vi "Check Adapter.vi"(8 "error in (no error)":errorcluster, 11 "Execution Service":refnum<class "Execution Service.lvclass">) -> (0 "error out":errorcluster, 3 "Adapter Loaded":bool)   [LabVIEW 2026, in "Execution Service.lvclass"]
uses:
  Execution Service.lvclass
  Execution Service.lvclass/Execution Service.ctl
  Interfaces/I Execution Adapter/I Execution Adapter.lvclass
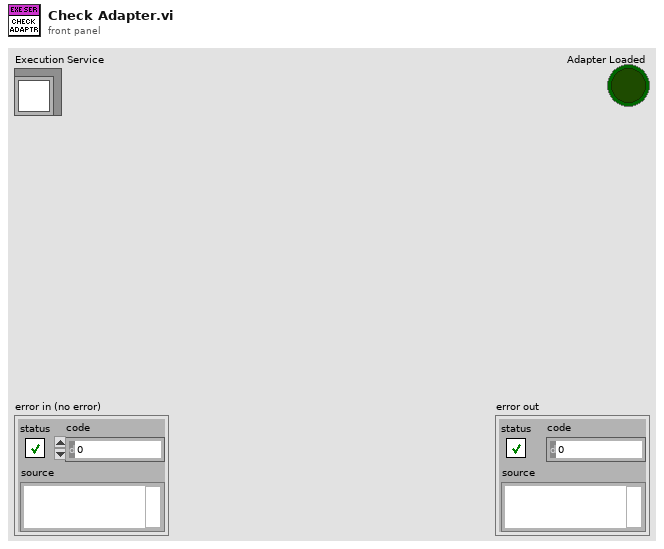
[diagram p1: front panel]
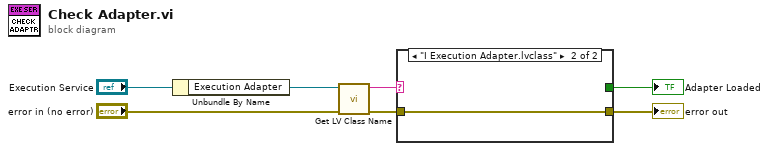
[diagram p0: block diagram]
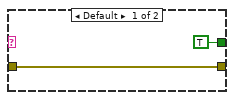
[diagram p2: hidden frame]
diagram:
  n1 = Unbundle By Name("Execution Service") -> ("Execution Adapter"=w5:refnum<class "I Execution Adapter.lvclass">)
  n2 = call <vilib>:"Get LV Class Name.vi"("error in (no error)"="error in (no error)", "object"=w5) -> ("error out"=w6:errorcluster, "class name"=w7:string)  [unwired: 8 in]
  n3 = case shown="\"I Execution Adapter.lvclass\"" w7 {
    tunnel: w6 -> [w8 w10]
    tunnel: [w8 w10] -> w2
    tunnel: [TRUE _] -> w1
    frame Default {
    }
    frame "I Execution Adapter.lvclass" {
    }
  }
  "error out" <- w2
  "Adapter Loaded" <- w1
